vi "Sign JWT.vi"(8 "error in (no error)":errorcluster, 9 "Key":string, 10 "Signature Algorithm":T1, 11 "JWT in":refnum<class "JWT.lvclass">) -> (0 "error out":errorcluster, 2 "JWT":string, 3 "JWT out":refnum<class "JWT.lvclass">)   [LabVIEW 2020, in "JWT.lvlib" / "JWT.lvclass"]
uses:
  JWT.lvclass
  JWT.lvlib
  Signature Algorithms.ctl
  lv-crypto/Crypto/Signature/Signature.lvclass
  lv-base64/Variant.ctl
  lv-base64/Base64.lvlib
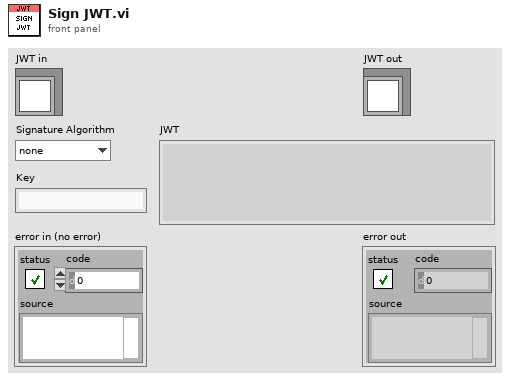
[diagram p1: front panel]
types:
  T1 = typedef "JWT.lvlib/Signature Algorithms.ctl" = enum16{"none", "HS256"}
  T2 = typedef "Base64.lvlib/Variant.ctl" = enum16{"Base64", "Base64-URL"}
  T3 = typedef "JWT.lvlib/JWT.lvclass/Additional Standard Claims.ctl" = cluster{"Issuer":string, "Subject":string, "Audience":string, "TokenID":string, "exp":timestamp, "nbf":timestamp, "iat":timestamp}
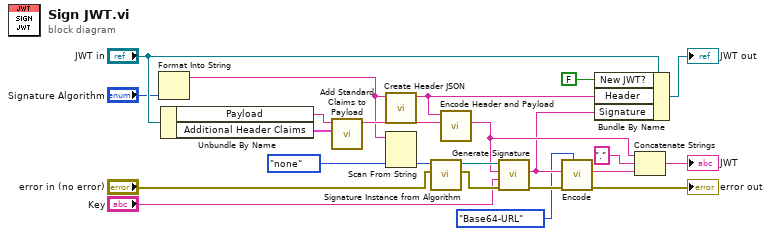
[diagram p0: block diagram]
diagram:
  n1 = Format Into String("Signature Algorithm") -> (resulting string=w1:string)  [unwired: 3 in, 1 out]
  n2 = Unbundle By Name("JWT in") -> ("Payload"=w9:string, "Additional Header Claims"=w10:T3)
  n3 = call "Add Standard Claims to Payload.vi"("Additional Standard Claims"=w10, "Payload JSON"=w9) -> ("Extended Payload"=w8:string)  [unwired: 9 in]
  n4 = call "Create Header JSON.vi"("alg"=w1) -> ("Header JSON"=w17:string)  [unwired: 9 in, 1 out]
  n5 = Scan From String(input string=w1, default 1=Signature_Algorithms."none" ("Signature Algorithm")) -> (output 1=w19:T1)  [unwired: 3 in, 3 out]
  n6 = call "Signature Instance from Algorithm.vi"("error in (no error)"="error in (no error)", "Signature Algorithm"=w19) -> ("error out"=w15:errorcluster, "Signature"=w16:refnum<class "Signature.lvclass">)  [unwired: 8 in]
  n7 = call "Encode Header and Payload.vi"("Payload"=w8, "Header"=w17) -> ("Encoded"=w14:string)  [unwired: 9 in]
  n8 = call-dynamic "Generate Signature.vi"("error in (no error)"=w15, "Key"="Key", "Message"=w14, "Signature in"=w16) -> ("error out"=w6:errorcluster, "Signature"=w7:string)  [unwired: 5 in, 1 out]
  n9 = call "Encode.vi"("Variant (Base64)"=Variant."Base64-URL", "error in (no error)"=w6, "string in (not encoded)"=w7) -> ("error out"=→"error out":errorcluster, "string out (base64-encoded)"=w4:string)  [unwired: 7 in]
  n10 = Bundle By Name(cluster="JWT in", "New JWT?"=FALSE, "Header"=w17, "Signature"=w7) -> (→"JWT out":refnum<class "JWT.lvclass">)
  n11 = Concatenate Strings(w14, "." ("string"), w4) -> (→"JWT":string)
